vi "Begin.vi"() -> (0 "error out":errorcluster)   [LabVIEW 2016]
doc: "Called before other user functions, this VI is expected to open initial I/O refnums, load in file data, and do all program initialization. Notice that the <B>error out</B> terminal is simply used for data flow. Wiring it to other structures or subVIs ensures that this VI runs first."
uses:
  <vilib>/Rock Robotics/WPI/DriverStation/WPI_DriverStationRobotMode2.ctl
  <vilib>/Rock Robotics/WPI/Joystick/WPI_JoystickDeviceEnum.ctl
  <vilib>/Rock Robotics/SystemInterfaces/AI/FPGA_AIChannel.ctl
  Drive/Drive Notifier.ctl
  Drive/Drive Control Type.ctl
  Intake/Intake Notifier.ctl
  Intake/Intake Control Type.ctl
  Climb/Climb Notifier.ctl
  Climb/Climb Control Type.ctl
  Rotation/Rotation Notifier.ctl
  Rotation/Rotation Control Type.ctl
  <vilib>/Rock Robotics/WPI/ThirdParty/CanMotor/TalonSRX/WPI_CANTalonSRX_APIControlMode.ctl
  <vilib>/Rock Robotics/WPI/ThirdParty/CanMotor/TalonSRX/WPI_CANTalonSRX_APIFeedbackSelect.ctl
  <vilib>/Rock Robotics/SystemInterfaces/DIO/FPGA_DIOPWMChannel.ctl
  <vilib>/Rock Robotics/SystemInterfaces/DIO/FPGA_DIOChannel.ctl
  Robot Global Data.vi
  Drive/Drive Globals.vi
  Intake/Intake Globals.vi
  Climb/Climb Globals.vi
  Rotation/Rotation Globals.vi
  <vilib>/Rock Robotics/WPI/MotorControl/WPI_MotorControlOpen Talon.vi
  <vilib>/Rock Robotics/WPI/ThirdParty/Sensors/Pigeon IMU/CTRE_PigeonIMU_Open_CAN.vi
  <vilib>/Rock Robotics/WPI/Counter/WPI_CounterDigitalInputToDigitalSource.vi
  <vilib>/Rock Robotics/WPI/Switch/WPI_SwitchOpenLimit.vi
  <vilib>/Rock Robotics/Network Tables/NT Write String.vi
panel:
  in  "error in":errorcluster
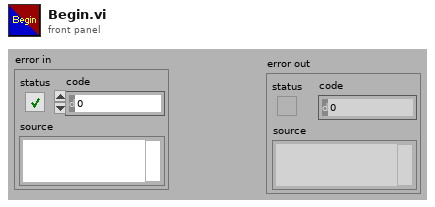
[diagram p1: front panel]
types:
  T1 = typedef "FPGA_DIOChannel.ctl" = enum8{"DIO 0", "DIO 1", "DIO 2", "DIO 3", "DIO 4", "DIO 5", "DIO 6", "DIO 7", "DIO 8", "DIO 9", "DIO MXP 0", "DIO MXP 1", "DIO MXP 2", "DIO MXP 3", "DIO MXP 4", "DIO MXP 5", "DIO MXP 6", "DIO MXP 7", "DIO MXP 8", "DIO MXP 9", "DIO MXP 10", "DIO MXP 11", "DIO MXP 12", "DIO MXP 13", "DIO MXP 14", "DIO MXP 15", "SPI Port CS1", "SPI Port CS2", "SPI Port CS3", "SPI Port MISO", "SPI Port MOSI", "Invalid"}
  T2 = typedef "WPI_JoystickDeviceEnum.ctl" = enum16{"USB 0", "USB 1", "USB 2", "USB 3", "USB 4", "USB 5"}
  T3 = typedef "FPGA_DIOPWMChannel.ctl" = enum8{"PWM 0", "PWM 1", "PWM 2", "PWM 3", "PWM 4", "PWM 5", "PWM 6", "PWM 7", "PWM 8", "PWM 9", "PWM MXP 0", "PWM MXP 1", "PWM MXP 2", "PWM MXP 3", "PWM MXP 4", "PWM MXP 5", "PWM MXP 6", "PWM MXP 7", "PWM MXP 8", "PWM MXP 9", "Invalid"}
  T4 = typedef "WPI_CANTalonSRX_APIFeedbackSelect.ctl" = enum16{"Digital Quadrature Encoder", "Analog Potentiometer", "Analog Encoder", "Count on Quad-A (Rising-Edge)", "Count on Quad-A (Falling-Edge)", "CTR Magnetic Enc (Absolute)", "CTR Magnetic Enc (Relative)", "Pulse Width"}
  T5 = typedef "WPI_CANTalonSRX_APIControlMode.ctl" = enum8{"Percent VBus", "Speed", "Position", "Slave", "Unchanged / Invalid", "Voltage Compensation", "Current", "Motion Profile", "Motion Magic"}
  T6 = typedef "Rotation Notifier.ctl" = cluster{"Up":bool, "Down":bool, "Rotation Control List":T7, "Control Down":bool, "Manual":bool, "Parameter 1":dbl, "Parameter 2":dbl, "Rotation Notifier":refnum<notifier>, "Step":i32}
  T7 = typedef "Rotation Control Type.ctl" = enum16{"No Op", "Up", "Down", "Control Up", "Control Down"}
  T8 = typedef "Climb Notifier.ctl" = cluster{"Up":bool, "Down":bool, "Climb Control List":T9}
  T9 = typedef "Climb Control Type.ctl" = enum16{"No Op", "Up", "Down"}
  T10 = typedef "Intake Notifier.ctl" = cluster{"In":bool, "Out":bool, "Intake Control List":T11, "Parameter 1":dbl, "Parameter 2":dbl, "Intake Notifier":refnum<notifier>, "Step":i32}
  T11 = typedef "Intake Control Type.ctl" = enum16{"No Op", "In", "Out"}
  T12 = typedef "Drive Notifier.ctl" = cluster{"Parameter 1":dbl, "Parameter 2":dbl, "Parameter 3":dbl, "Drive Control List":T13, "Parameter 4":dbl, "Gear Angle":dbl, "Parameter 6":dbl, "Parameter 7":dbl, "Parameter 8":dbl, "Parameter 9":dbl, "Robotcentric":bool, "Reset Gyro":bool, "Reset Wheels":bool, "Turn to Gear Left":bool, "Turn to Gear Center":bool, "Turn to Gear Right":bool, "Half Power":bool, "Drive Notifier":refnum<notifier>, "Step":i32}
  T13 = typedef "Drive Control Type.ctl" = enum16{"No Op", "Fieldcentric", "Robotcentric", "Reset Wheel Position", "Reset Gyro Value", "Turn to Angle", "Drive For Time"}
  T14 = typedef "FPGA_AIChannel.ctl" = enum8{"AI 0", "AI 1", "AI 2", "AI 3", "AI MXP 0", "AI MXP 1", "AI MXP 2", "AI MXP 3", "Invalid"}
  T15 = typedef "WPI_DriverStationRobotMode2.ctl" = enum16{"Autonomous Disabled", "Autonomous Enabled", "Teleop Disabled", "Teleop Enabled", "Disconnected", "Finish", "Test Disabled", "Test Enabled", "Emergency Stopped"}
  T16 = typedef "WPI_JoystickDevRef.ctl" = cluster{"Device":T2}
  T17 = typedef "WPI_MotorControlDeviceRef.ctl" = cluster{"DeviceStatus":errorcluster, "Type":T18, "PWM":cluster{"PWM Channel":T3, "DeadBand":T19}, "CAN":cluster{"Device Number":u8, "SetOutput VI Ref":variant, "GetOutput VI Ref":variant, "Enable VI Ref":variant, "Disable VI Ref":variant, "Data":variant}, "Invert":bool}
  T18 = typedef "WPI_MotorControlType.ctl" = enum16{"PWM", "CAN"}
  T19 = typedef "WPI_PWMDeadband.ctl" = cluster{"Name":string, "maxPositivePwm":i32, "minPositivePwm":i32, "centerPwm":i32, "maxNegativePwm":i32, "minNegativePwm":i32, "angularRange":u16}
  T20 = typedef "WPI_DigitalInputDevRef.ctl" = cluster{"DevStatus":errorcluster, "DIO Channel":T1}
  T21 = typedef "CTRE_PigeonIMU_DeviceRef.ctl" = cluster{"DeviceStatus":errorcluster, "Device Number":u8, "Type":T22, "Device ID":u32}
  T22 = typedef "CTRE_PigeonIMU_ConnectionType.ctl" = u32
  T23 = typedef "FPGA_CounterEncoderSourceConvertionLVSourceType.ctl" = cluster{"DevStatus":errorcluster, "AnalogTriggerMode?":bool, "DigitalMode":cluster{"DIO Channel":T24}, "AnalogTriggerMode":cluster{"AnalogTriggerIndex":T25, "OutputType":T26}}
  T24 = typedef "FPGA_DIODigitalSourceChannel.ctl" = enum8{"DIO 0", "DIO 1", "DIO 2", "DIO 3", "DIO 4", "DIO 5", "DIO 6", "DIO 7", "DIO 8", "DIO 9", "DIO MXP 0", "DIO MXP 1", "DIO MXP 2", "DIO MXP 3", "DIO MXP 4", "DIO MXP 5", "DIO MXP 6", "DIO MXP 7", "DIO MXP 8", "DIO MXP 9", "DIO MXP 10", "DIO MXP 11", "DIO MXP 12", "DIO MXP 13", "DIO MXP 14", "DIO MXP 15", "Disabled"}
  T25 = typedef "FPGA_AnalogTriggerIndex.ctl" = enum8{"Trig 0", "Trig 1", "Trig 2", "Trig 3", "Trig 4", "Trig 5", "Trig 6", "Trig 7", "Invalid"}
  T26 = typedef "FPGA_AnalogTriggerOutType.ctl" = enum16{"InWindow", "TriggerState", "Rising", "Falling"}
  T27 = typedef "WPI_EncoderDevRef.ctl" = cluster{"DevStatus":errorcluster, "EncoderIndex":T28, "CounterIndex":T29, "DistancePerCount":dbl, "Decoding Type":T30}
  T28 = typedef "FPGA_EncoderIdx.ctl" = enum8{"Enc 0", "Enc 1", "Enc 2", "Enc 3", "Enc 4", "Enc 5", "Enc 6", "Enc 7", "Invalid"}
  T29 = typedef "FPGA_CounterCtrSystemIndex.ctl" = enum8{"Ctr 0", "Ctr 1", "Ctr 2", "Ctr 3", "Ctr 4", "Ctr 5", "Ctr 6", "Ctr 7", "Invalid"}
  T30 = typedef "WPI_EncoderType.ctl" = enum16{"1x", "2x", "4x"}
  T31 = typedef "WPI_AnalogChannelDevRef.ctl" = cluster{"DevStatus":errorcluster, "Analog Channel":T14}
  T32 = typedef "WPI_SwitchDevRef.ctl" = cluster{"DevStatus":errorcluster, "DIO Channel":T1, "CntIndex":T29, "Normally Closed":bool}
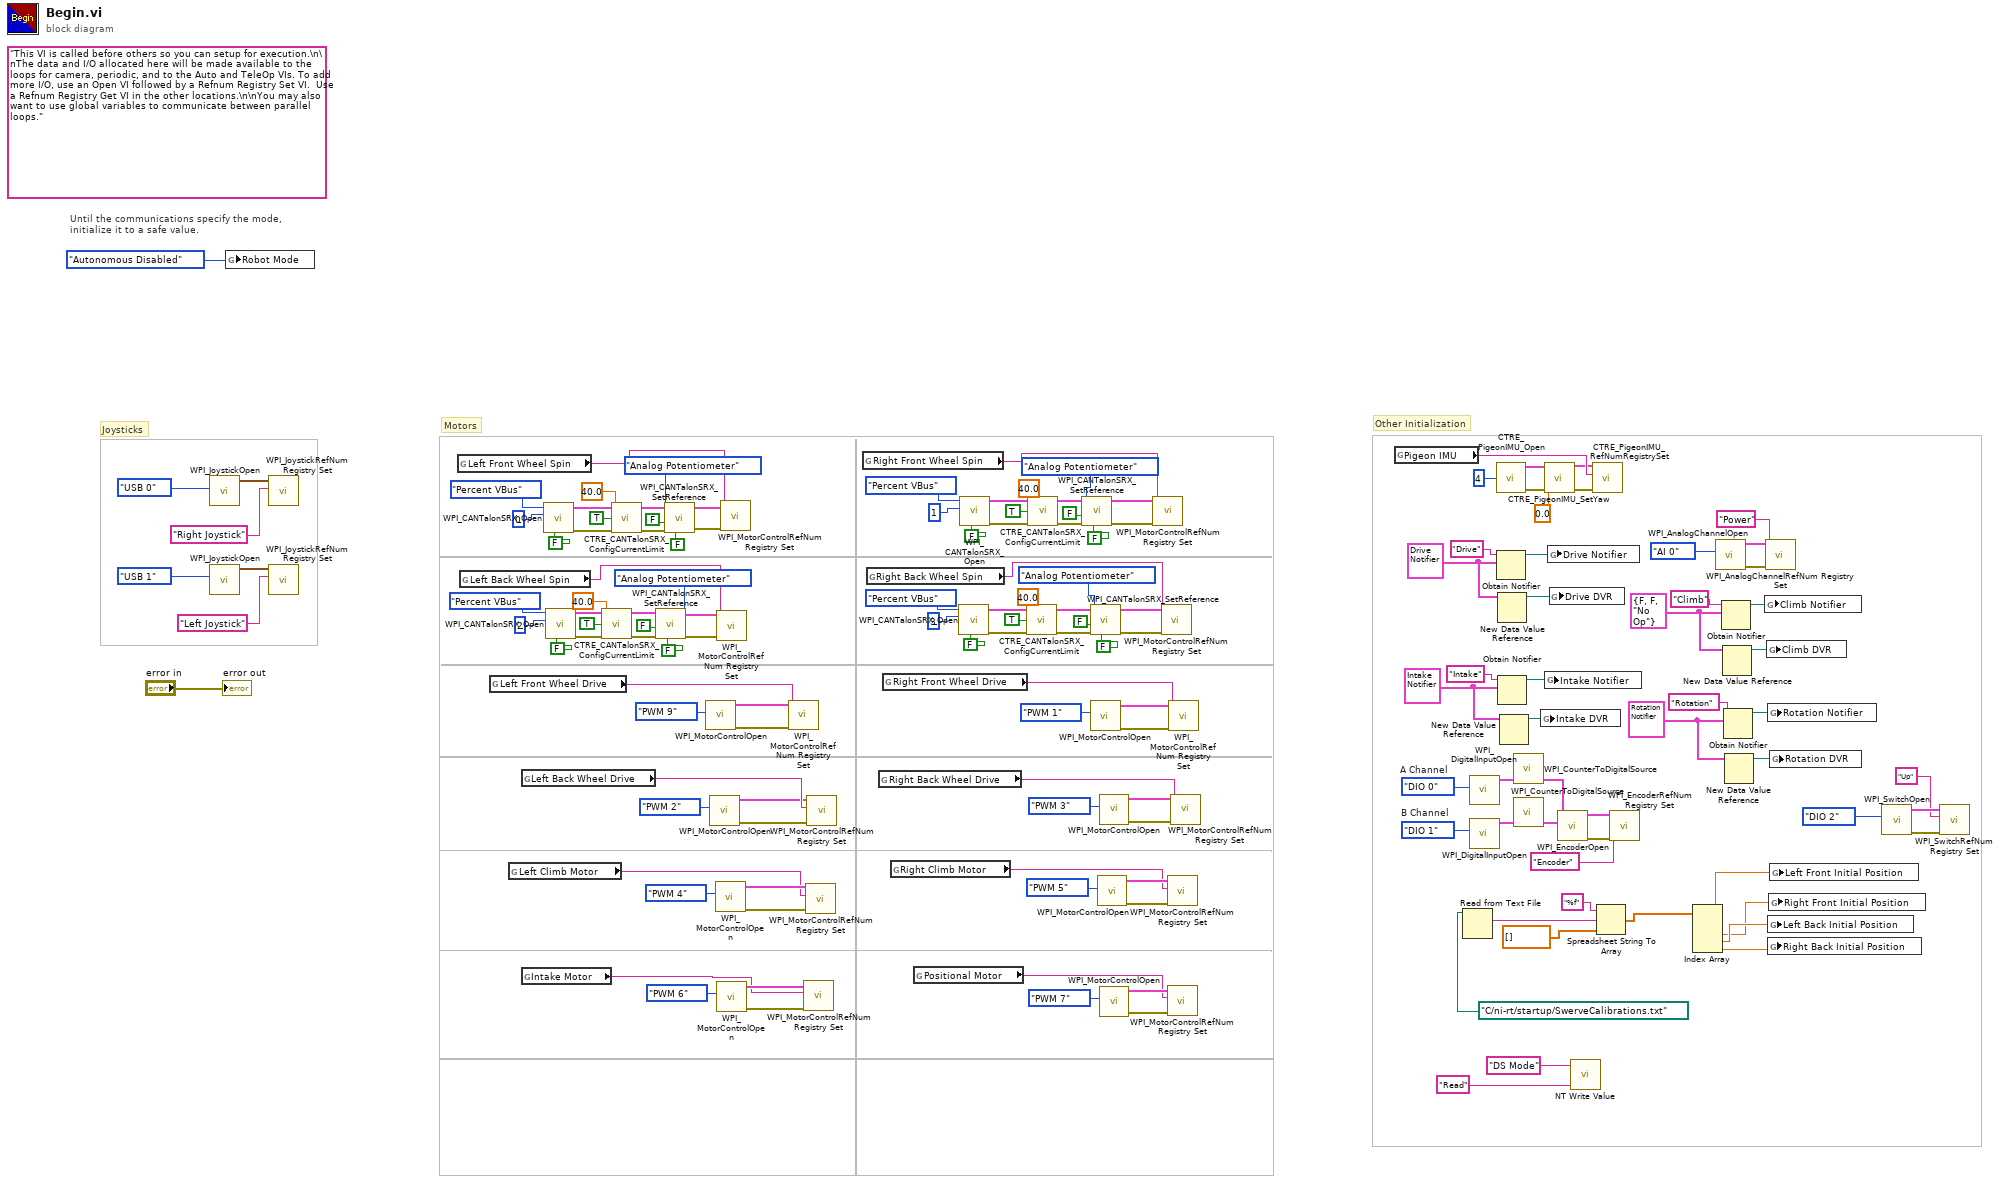
[diagram p0: block diagram]
diagram:
  w24 = FPGA_DIOChannel."DIO 1"  # B Channel
  w23 = FPGA_DIOChannel."DIO 0"  # A Channel
  w129 = T6 {"Up"=FALSE, "Down"=FALSE, "Rotation Control List"=enum."No Op", "Control Down"=FALSE, "Manual"=FALSE, "Parameter 1"=0.0, "Parameter 2"=0.0, "Rotation Notifier"=refnum, "Step"=0} ("Rotation Notifier")
  w133 = T8 {"Up"=FALSE, "Down"=FALSE, "Climb Control List"=enum."No Op"} ("Intake Notifier")
  w139 = T10 {"In"=FALSE, "Out"=FALSE, "Intake Control List"=enum."No Op", "Parameter 1"=0.0, "Parameter 2"=0.0, "Intake Notifier"=refnum, "Step"=0} ("Intake Notifier")
  w140 = T12 {"Parameter 1"=0.0, "Parameter 2"=0.0, "Parameter 3"=0.0, "Drive Control List"=enum."No Op", "Parameter 4"=0.0, "Gear Angle"=0.0, "Parameter 6"=0.0, "Parameter 7"=0.0, "Parameter 8"=0.0, "Parameter 9"=0.0, "Robotcentric"=FALSE, "Reset Gyro"=FALSE, "Reset Wheels"=FALSE, "Turn to Gear Left"=FALSE, "Turn to Gear Center"=FALSE, "Turn to Gear Right"=FALSE, "Half Power"=FALSE, "Drive Notifier"=refnum, "Step"=0} ("Drive Notifier")
  (unwired) "This VI is called before others so you can setup for execution.\n\nThe data and I/O allocated here will be made available to the loops for camera, periodic, and to the Auto and TeleOp VIs. To add more I/O, use an Open VI followed by a Refnum Registry Set VI.  Use a Refnum Registry Get VI in the other locations.\n\nYou may also want to use global variables to communicate between parallel loops."
  # "Motors"
  # "Other Initialization"
  # "Joysticks"
  # "Until the communications specify the mode,\ninitialize it to a safe value."
  n1 = call <vilib>:"WPI_JoystickOpen.vi"("JoystickDevice"=WPI_JoystickDeviceEnum."USB 0") -> ("JoystickDevRef"=w149:T16)  [unwired: 10 in]
  n2 = call <vilib>:"WPI_JoystickOpen.vi"("JoystickDevice"=WPI_JoystickDeviceEnum."USB 1") -> ("JoystickDevRef"=w26:T16)  [unwired: 10 in]
  n3 = global write "Robot Global Data.vi" "Robot Mode"(WPI_DriverStationRobotMode2."Autonomous Disabled" ("Robot Mode")) -> ()
  n4 = call <vilib>:"WPI_JoystickRefNum Registry Set.vi"("refnum name"="Right Joystick", "JoystickDevRef"=w149) -> ()  [unwired: 8 in, 2 out]
  n5 = call <vilib>:"WPI_JoystickRefNum Registry Set.vi"("refnum name"="Left Joystick", "JoystickDevRef"=w26) -> ()  [unwired: 8 in, 2 out]
  n6 = global read "Drive Globals.vi" "Left Front Wheel Spin"() -> (w79:string)
  n7 = global read "Drive Globals.vi" "Left Back Wheel Spin"() -> (w80:string)
  n8 = global read "Drive Globals.vi" "Left Front Wheel Drive"() -> (w81:string)
  n9 = global read "Climb Globals.vi" "Left Climb Motor"() -> (w48:string)
  n10 = global read "Drive Globals.vi" "Left Back Wheel Drive"() -> (w76:string)
  n11 = global read "Intake Globals.vi" "Intake Motor"() -> (w47:string)
  n12 = call <vilib>:"WPI_CANTalonSRX_Open.vi"("Invert"=FALSE, "Device Number"=u8 0, "Control Mode"=WPI_CANTalonSRX_APIControlMode."Percent VBus") -> ("error out"=w120:errorcluster, "CAN Talon SRX Ref"=w119:T17)  [unwired: 7 in]
  n13 = call <vilib>:"WPI_CANTalonSRX_Open.vi"("Invert"=FALSE, "Device Number"=u8 2, "Control Mode"=WPI_CANTalonSRX_APIControlMode."Percent VBus") -> ("error out"=w109:errorcluster, "CAN Talon SRX Ref"=w110:T17)  [unwired: 7 in]
  n14 = call <vilib>:"CTRE_CANTalonSRX_ConfigCurrentLimit.vi"("error in (no error)"=w109, "Enable Current Limit?"=TRUE, "Current Limit (Amps)"=40.0, "CAN Talon SRX Ref"=w110) -> ("error out"=w111:errorcluster, "CAN Talon SRX Ref"=w112:T17)  [unwired: 6 in]
  n15 = call <vilib>:"CTRE_CANTalonSRX_ConfigCurrentLimit.vi"("error in (no error)"=w120, "Enable Current Limit?"=TRUE, "Current Limit (Amps)"=40.0, "CAN Talon SRX Ref"=w119) -> ("error out"=w118:errorcluster, "CAN Talon SRX Ref"=w117:T17)  [unwired: 6 in]
  n16 = call <vilib>:"WPI_CANTalonSRX_SetReference.vi"("Reverse Closed-Loop Output"=FALSE, "error in (no error)"=w111, "Reverse Feedback Sensor"=FALSE, "Feedback Reference"=WPI_CANTalonSRX_APIFeedbackSelect."Analog Potentiometer", "CAN Talon SRX Ref"=w112) -> ("error out"=w34:errorcluster, "CAN Talon SRX Ref"=w35:T17)  [unwired: 5 in]
  n17 = call <vilib>:"WPI_CANTalonSRX_SetReference.vi"("Reverse Closed-Loop Output"=FALSE, "error in (no error)"=w118, "Reverse Feedback Sensor"=FALSE, "Feedback Reference"=WPI_CANTalonSRX_APIFeedbackSelect."Analog Potentiometer", "CAN Talon SRX Ref"=w117) -> ("error out"=w28:errorcluster, "CAN Talon SRX Ref"=w29:T17)  [unwired: 5 in]
  n18 = call-poly <vilib>:"WPI_MotorControlOpen.vi"("PWM Channel"=FPGA_DIOPWMChannel."PWM 9") -> ("error out"=w70:errorcluster, "MotorControlDeviceRef"=w71:T17)  [unwired: 9 in]
  n19 = call-poly <vilib>:"WPI_MotorControlOpen.vi"("PWM Channel"=FPGA_DIOPWMChannel."PWM 2") -> ("error out"=w73:errorcluster, "MotorControlDeviceRef"=w72:T17)  [unwired: 9 in]
  n20 = call-poly <vilib>:"WPI_MotorControlOpen.vi"("PWM Channel"=FPGA_DIOPWMChannel."PWM 4") -> ("error out"=w56:errorcluster, "MotorControlDeviceRef"=w57:T17)  [unwired: 9 in]
  n21 = call <vilib>:"WPI_MotorControlRefNum Registry Set.vi"("error in (no error)"=w34, "refnum name"=w80, "MotorControlDevRef"=w35) -> ()  [unwired: 7 in, 2 out]
  n22 = call-poly <vilib>:"WPI_MotorControlOpen.vi"("PWM Channel"=FPGA_DIOPWMChannel."PWM 6") -> ("error out"=w54:errorcluster, "MotorControlDeviceRef"=w55:T17)  [unwired: 9 in]
  n23 = call <vilib>:"WPI_MotorControlRefNum Registry Set.vi"("error in (no error)"=w28, "refnum name"=w79, "MotorControlDevRef"=w29) -> ()  [unwired: 7 in, 2 out]
  n24 = call <vilib>:"WPI_MotorControlRefNum Registry Set.vi"("error in (no error)"=w70, "refnum name"=w81, "MotorControlDevRef"=w71) -> ()  [unwired: 7 in, 2 out]
  n25 = call <vilib>:"WPI_MotorControlRefNum Registry Set.vi"("error in (no error)"=w54, "refnum name"=w47, "MotorControlDevRef"=w55) -> ()  [unwired: 7 in, 2 out]
  n26 = call <vilib>:"WPI_MotorControlRefNum Registry Set.vi"("error in (no error)"=w56, "refnum name"=w48, "MotorControlDevRef"=w57) -> ()  [unwired: 7 in, 2 out]
  n27 = call <vilib>:"WPI_MotorControlRefNum Registry Set.vi"("error in (no error)"=w73, "refnum name"=w76, "MotorControlDevRef"=w72) -> ()  [unwired: 7 in, 2 out]
  n28 = global read "Drive Globals.vi" "Right Front Wheel Spin"() -> (w78:string)
  n29 = global read "Drive Globals.vi" "Right Back Wheel Spin"() -> (w77:string)
  n30 = global read "Drive Globals.vi" "Right Back Wheel Drive"() -> (w74:string)
  n31 = global read "Drive Globals.vi" "Right Front Wheel Drive"() -> (w75:string)
  n32 = global read "Climb Globals.vi" "Right Climb Motor"() -> (w49:string)
  n33 = global read "Rotation Globals.vi" "Positional Motor"() -> (w46:string)
  n34 = call <vilib>:"WPI_CANTalonSRX_Open.vi"("Invert"=FALSE, "Device Number"=u8 3, "Control Mode"=WPI_CANTalonSRX_APIControlMode."Percent VBus") -> ("error out"=w98:errorcluster, "CAN Talon SRX Ref"=w97:T17)  [unwired: 7 in]
  n35 = call <vilib>:"WPI_CANTalonSRX_Open.vi"("Invert"=FALSE, "Device Number"=u8 1, "Control Mode"=WPI_CANTalonSRX_APIControlMode."Percent VBus") -> ("error out"=w87:errorcluster, "CAN Talon SRX Ref"=w88:T17)  [unwired: 7 in]
  n36 = call <vilib>:"CTRE_CANTalonSRX_ConfigCurrentLimit.vi"("error in (no error)"=w98, "Enable Current Limit?"=TRUE, "Current Limit (Amps)"=40.0, "CAN Talon SRX Ref"=w97) -> ("error out"=w96:errorcluster, "CAN Talon SRX Ref"=w95:T17)  [unwired: 6 in]
  n37 = call <vilib>:"CTRE_CANTalonSRX_ConfigCurrentLimit.vi"("error in (no error)"=w87, "Enable Current Limit?"=TRUE, "Current Limit (Amps)"=40.0, "CAN Talon SRX Ref"=w88) -> ("error out"=w89:errorcluster, "CAN Talon SRX Ref"=w90:T17)  [unwired: 6 in]
  n38 = call <vilib>:"WPI_CANTalonSRX_SetReference.vi"("Reverse Closed-Loop Output"=FALSE, "error in (no error)"=w89, "Reverse Feedback Sensor"=FALSE, "Feedback Reference"=WPI_CANTalonSRX_APIFeedbackSelect."Analog Potentiometer", "CAN Talon SRX Ref"=w90) -> ("error out"=w30:errorcluster, "CAN Talon SRX Ref"=w31:T17)  [unwired: 5 in]
  n39 = call <vilib>:"WPI_CANTalonSRX_SetReference.vi"("Reverse Closed-Loop Output"=FALSE, "error in (no error)"=w96, "Reverse Feedback Sensor"=FALSE, "Feedback Reference"=WPI_CANTalonSRX_APIFeedbackSelect."Analog Potentiometer", "CAN Talon SRX Ref"=w95) -> ("error out"=w32:errorcluster, "CAN Talon SRX Ref"=w33:T17)  [unwired: 5 in]
  n40 = call-poly <vilib>:"WPI_MotorControlOpen.vi"("PWM Channel"=FPGA_DIOPWMChannel."PWM 1") -> ("error out"=w69:errorcluster, "MotorControlDeviceRef"=w68:T17)  [unwired: 9 in]
  n41 = call-poly <vilib>:"WPI_MotorControlOpen.vi"("PWM Channel"=FPGA_DIOPWMChannel."PWM 5") -> ("error out"=w50:errorcluster, "MotorControlDeviceRef"=w51:T17)  [unwired: 9 in]
  n42 = call-poly <vilib>:"WPI_MotorControlOpen.vi"("PWM Channel"=FPGA_DIOPWMChannel."PWM 3") -> ("error out"=w67:errorcluster, "MotorControlDeviceRef"=w66:T17)  [unwired: 9 in]
  n43 = call-poly <vilib>:"WPI_MotorControlOpen.vi"("PWM Channel"=FPGA_DIOPWMChannel."PWM 7") -> ("error out"=w52:errorcluster, "MotorControlDeviceRef"=w53:T17)  [unwired: 9 in]
  n44 = call <vilib>:"WPI_MotorControlRefNum Registry Set.vi"("error in (no error)"=w30, "refnum name"=w78, "MotorControlDevRef"=w31) -> ()  [unwired: 7 in, 2 out]
  n45 = call <vilib>:"WPI_MotorControlRefNum Registry Set.vi"("error in (no error)"=w32, "refnum name"=w77, "MotorControlDevRef"=w33) -> ()  [unwired: 7 in, 2 out]
  n46 = call <vilib>:"WPI_MotorControlRefNum Registry Set.vi"("error in (no error)"=w50, "refnum name"=w49, "MotorControlDevRef"=w51) -> ()  [unwired: 7 in, 2 out]
  n47 = call <vilib>:"WPI_MotorControlRefNum Registry Set.vi"("error in (no error)"=w52, "refnum name"=w46, "MotorControlDevRef"=w53) -> ()  [unwired: 7 in, 2 out]
  n48 = call <vilib>:"WPI_MotorControlRefNum Registry Set.vi"("error in (no error)"=w69, "refnum name"=w75, "MotorControlDevRef"=w68) -> ()  [unwired: 7 in, 2 out]
  n49 = call <vilib>:"WPI_MotorControlRefNum Registry Set.vi"("error in (no error)"=w67, "refnum name"=w74, "MotorControlDevRef"=w66) -> ()  [unwired: 7 in, 2 out]
  n50 = global read "Drive Globals.vi" "Pigeon IMU"() -> (w44:string)
  n51 = Read from Text File(file (use dialog)=path "C:/ni-rt/startup/SwerveCalibrations.txt") -> (text=w15:string)  [unwired: 3 in, 3 out]
  n52 = call <vilib>:"WPI_DigitalInputOpen.vi"("DIO Channel"=w23) -> ("DigitalInputDevRef"=w20:T20)  [unwired: 1 in, 9 out]
  n53 = call <vilib>:"WPI_DigitalInputOpen.vi"("DIO Channel"=w24) -> ("DigitalInputDevRef"=w21:T20)  [unwired: 1 in, 9 out]
  n54 = call-poly <vilib>:"CTRE_PigeonIMU_Open.vi"("Device Number"=u8 4) -> ("error out"=w37:errorcluster, "PigeonIMUDevRef"=w40:T21)  [unwired: 9 in]
  n55 = Obtain Notifier(name (unnamed)="Drive", notification data type=w140) -> (notifier out=w138:refnum<notifier>)  [unwired: 2 in, 2 out]
  n56 = New Data Value Reference(data value=w140) -> (data value reference=w137:refnum<data-value>)  [unwired: 1 in, 1 out]
  n57 = Obtain Notifier(name (unnamed)="Intake", notification data type=w139) -> (notifier out=w136:refnum<notifier>)  [unwired: 2 in, 2 out]
  n58 = New Data Value Reference(data value=w139) -> (data value reference=w135:refnum<data-value>)  [unwired: 1 in, 1 out]
  n59 = call-poly <vilib>:"WPI_CounterToDigitalSource.vi"("DigitalInputDevRef"=w20) -> ("Digital Source"=w19:T23)  [unwired: 6 out]
  n60 = call-poly <vilib>:"WPI_CounterToDigitalSource.vi"("DigitalInputDevRef"=w21) -> ("Digital Source"=w22:T23)  [unwired: 6 out]
  n61 = global write "Intake Globals.vi" "Intake DVR"(w135) -> ()
  n62 = call <vilib>:"CTRE_PigeonIMU_SetYaw.vi"("error in (no error)"=w37, "Value"=0.0, "PigeonIMUDevRef"=w40) -> ("error out"=w38:errorcluster, "PigeonIMUDevRef"=w39:T21)  [unwired: 7 in]
  n63 = global write "Intake Globals.vi" "Intake Notifier"(w136) -> ()
  n64 = global write "Drive Globals.vi" "Drive Notifier"(w138) -> ()
  n65 = global write "Drive Globals.vi" "Drive DVR"(w137) -> ()
  n66 = call <vilib>:"WPI_EncoderOpen.vi"("BSource"=w22, "ASource"=w19) -> ("error out"=w18:errorcluster, "EncoderDevRef"=w17:T27)  [unwired: 6 in, 2 out]
  n67 = call-poly <vilib>:"NT Write Value.vi"("String"="Read", "Name"="DS Mode") -> ()  [unwired: 9 in, 1 out]
  n68 = call <vilib>:"CTRE_PigeonIMU_RefNumRegistrySet.vi"("error in (no error)"=w38, "refnum name"=w44, "PigeonIMUDevRef"=w39) -> ()  [unwired: 7 in, 2 out]
  n69 = Spreadsheet String To Array(format string="%f", spreadsheet string=w15, array type (2D Dbl)=dbl[] []) -> (array=w13:dbl[])  [unwired: 1 in]
  n70 = call <vilib>:"WPI_EncoderRefNum Registry Set.vi"("error in (no error)"=w18, "refnum name"="Encoder", "EncoderDevRef"=w17) -> ()  [unwired: 7 in, 2 out]
  n71 = Index Array(array=w13) -> (element #1=w8:dbl, element #2=w9:dbl, element #3=w10:dbl, element #4=w11:dbl)  [unwired: 4 in]
  n72 = call <vilib>:"WPI_AnalogChannelOpen.vi"("Analog Channel"=FPGA_AIChannel."AI 0") -> ("error out"=w144:errorcluster, "AIDeviceRef"=w143:T31)  [unwired: 9 in]
  n73 = Obtain Notifier(name (unnamed)="Climb", notification data type=w133) -> (notifier out=w132:refnum<notifier>)  [unwired: 2 in, 2 out]
  n74 = New Data Value Reference(data value=w133) -> (data value reference=w131:refnum<data-value>)  [unwired: 1 in, 1 out]
  n75 = Obtain Notifier(name (unnamed)="Rotation", notification data type=w129) -> (notifier out=w128:refnum<notifier>)  [unwired: 2 in, 2 out]
  n76 = New Data Value Reference(data value=w129) -> (data value reference=w127:refnum<data-value>)  [unwired: 1 in, 1 out]
  n77 = global write "Climb Globals.vi" "Climb Notifier"(w132) -> ()
  n78 = call <vilib>:"WPI_AnalogChannelRefNum Registry Set.vi"("error in (no error)"=w144, "refnum name"="Power", "AIDeviceRef"=w143) -> ()  [unwired: 7 in, 2 out]
  n79 = global write "Climb Globals.vi" "Climb DVR"(w131) -> ()
  n80 = global write "Rotation Globals.vi" "Rotation Notifier"(w128) -> ()
  n81 = global write "Drive Globals.vi" "Left Back Initial Position"(w10) -> ()
  n82 = global write "Drive Globals.vi" "Right Back Initial Position"(w11) -> ()
  n83 = global write "Drive Globals.vi" "Right Front Initial Position"(w9) -> ()
  n84 = global write "Rotation Globals.vi" "Rotation DVR"(w127) -> ()
  n85 = global write "Drive Globals.vi" "Left Front Initial Position"(w8) -> ()
  n86 = call-poly <vilib>:"WPI_SwitchOpen.vi"("DIO Channel"=FPGA_DIOChannel."DIO 2") -> ("error out"=w4:errorcluster, "SwitchDevRef"=w5:T32)  [unwired: 9 in]
  n87 = call <vilib>:"WPI_SwitchRefNum Registry Set.vi"("error in (no error)"=w4, "refnum name"="Up", "SwitchDevRef"=w5) -> ()  [unwired: 7 in, 2 out]
  "error out" <- "error in"
